vi "Funct acq pre-checks-obtain items to copy.vi"(11 "Experiment folder path":path) -> (0 "error out":errorcluster, 3 "Files and folders to copy":string[](array[string]))   [LabVIEW 2013]
uses:
  Program Files (x86)/National Instruments/LabVIEW 2013/user.lib/_OpenG.lib/array/array.llb/Search 1D Array (String)__ogtk.vi
  Program Files (x86)/National Instruments/LabVIEW 2013/user.lib/_OpenG.lib/array/array.llb/Delete Elements from 1D Array (String)__ogtk.vi
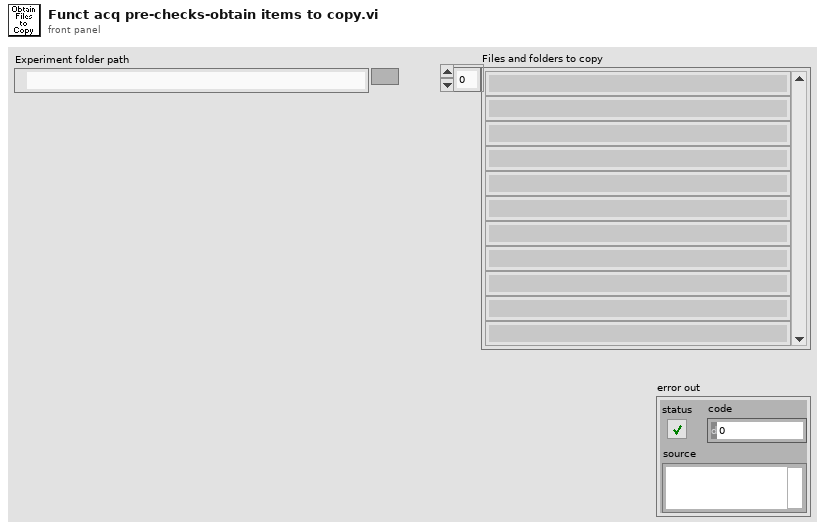
[diagram p1: front panel]
types:
  T1 = typedef "Fixed strings.ctl" = cluster{"ROI file name":string, "Normalised ROI file name":string, "Zplane Pockels values file name":string, "Functional data folder name":string, "Experiment Header file name":string, "Z-stack images folder name":string, "Groups setup rel. path":string, "Groups text file rel. path":string, "TDMS files folder name (F.img)":string, "TDMS files folder name (V.acq)":string, "TDMS files folder name (Pl.acq)":string, "Cycle rel times sequence file":string, "Dynamically called VIs folder name":string, "Time Series folder base name":string}
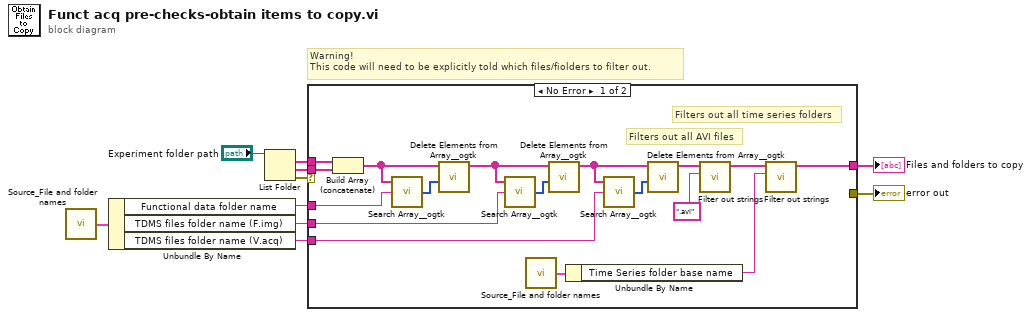
[diagram p0: block diagram]
diagram:
  # "Warning!\nThis code will need to be explicitly told which files/fiolders to filter out."
  n1 = call "Source_File and folder names.vi"() -> ("Fixed strings"=w10:T1)  [unwired: 1 in]
  n2 = Unbundle By Name(w10) -> ("Functional data folder name"=w6:string, "TDMS files folder name (F.img)"=w4:string, "TDMS files folder name (V.acq)"=w1:string)
  n3 = List Folder(path="Experiment folder path") -> (filenames=w8:string[], folder names=w9:string[], error out=w3:errorcluster)  [unwired: 3 in, 1 out]
  n4 = case shown="No Error" w3 {
    selector: w3 -> [_ w28]
    tunnel: w9 -> [w27 _]
    tunnel: w8 -> [w26 _]
    tunnel: w6 -> [w23 _]
    tunnel: [w16 _] -> w5
    tunnel: w4 -> [w21 _]
    tunnel: [_ w28] -> w2
    tunnel: w1 -> [w11 _]
    frame No Error {
      # "Filters out all time series folders"
      # "Filters out all AVI files"
      n5 = Build Array (concatenate)(w26, w27) -> (w25:string[])
      n6 = call-poly "Search Array__ogtk.vi"("Array"=w25, "Element Data"=w23) -> ("Indices of Elements"=w24:i32[])  [unwired: 7 in]
      n7 = call-poly "Delete Elements from Array__ogtk.vi"("indices"=w24, "array"=w25) -> ("array w/ subset deleted"=w20:string[])  [unwired: 8 in, 1 out]
      n8 = call-poly "Search Array__ogtk.vi"("Array"=w20, "Element Data"=w21) -> ("Indices of Elements"=w22:i32[])  [unwired: 7 in]
      n9 = call "Source_File and folder names.vi"() -> ("Fixed strings"=w18:T1)  [unwired: 1 in]
      n10 = call-poly "Delete Elements from Array__ogtk.vi"("indices"=w22, "array"=w20) -> ("array w/ subset deleted"=w13:string[])  [unwired: 8 in, 1 out]
      n11 = Unbundle By Name(w18) -> ("Time Series folder base name"=w15:string)
      n12 = call-poly "Search Array__ogtk.vi"("Array"=w13, "Element Data"=w11) -> ("Indices of Elements"=w14:i32[])  [unwired: 7 in]
      n13 = call-poly "Delete Elements from Array__ogtk.vi"("indices"=w14, "array"=w13) -> ("array w/ subset deleted"=w12:string[])  [unwired: 8 in, 1 out]
      n14 = call "Filter out strings.vi"("Filter out if containing this string"=".avi", "array w/ subset deleted in"=w12) -> ("array w/ subset deleted out"=w17:string[])  [unwired: 9 in]
      n15 = call "Filter out strings.vi"("Filter out if containing this string"=w15, "array w/ subset deleted in"=w17) -> ("array w/ subset deleted out"=w16:string[])  [unwired: 9 in]
    }
    frame Error {
    }
  }
  "Files and folders to copy" <- w5
  "error out" <- w2
